vi "THETA_2.vi"(8 "error in (no error)":errorcluster, 11 "reference in":refnum<class "Manipulator.lvclass">) -> (0 "error out":errorcluster, 3 "reference out":refnum<class "Manipulator.lvclass">)   [LabVIEW 2014, in "Manipulator.lvclass"]
uses:
  Manipulator.lvclass
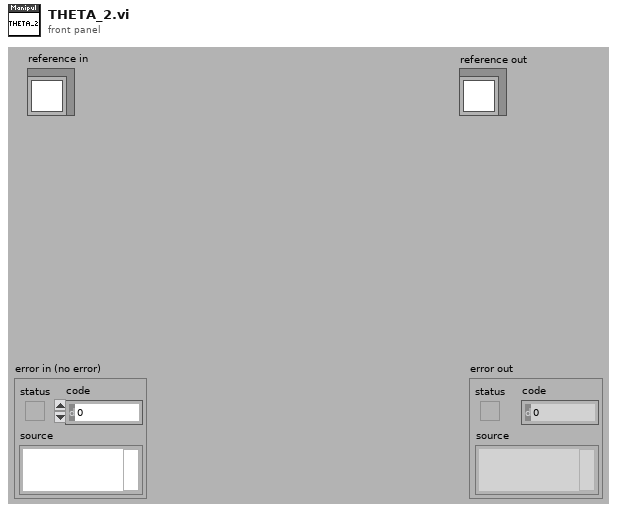
[diagram p1: front panel]
types:
  T1 = typedef "Manipulator.lvclass/ObjectAttributes.ctl" = cluster{"Coordinates":cluster{"X":dbl, "Y":dbl, "Z":dbl}, "Angles":cluster{"THETA_1":dbl, "THETA_2":dbl, "THETA_3":dbl, "THETA_4":dbl, "THETA_5":dbl, "THETA_6":dbl, "THETA_7":dbl, "THETA_8":dbl, "THETA_9":dbl, "THETA_10":dbl}, "Lengths":cluster{"a":dbl, "b":dbl, "c":dbl, "d":dbl, "e":dbl}}
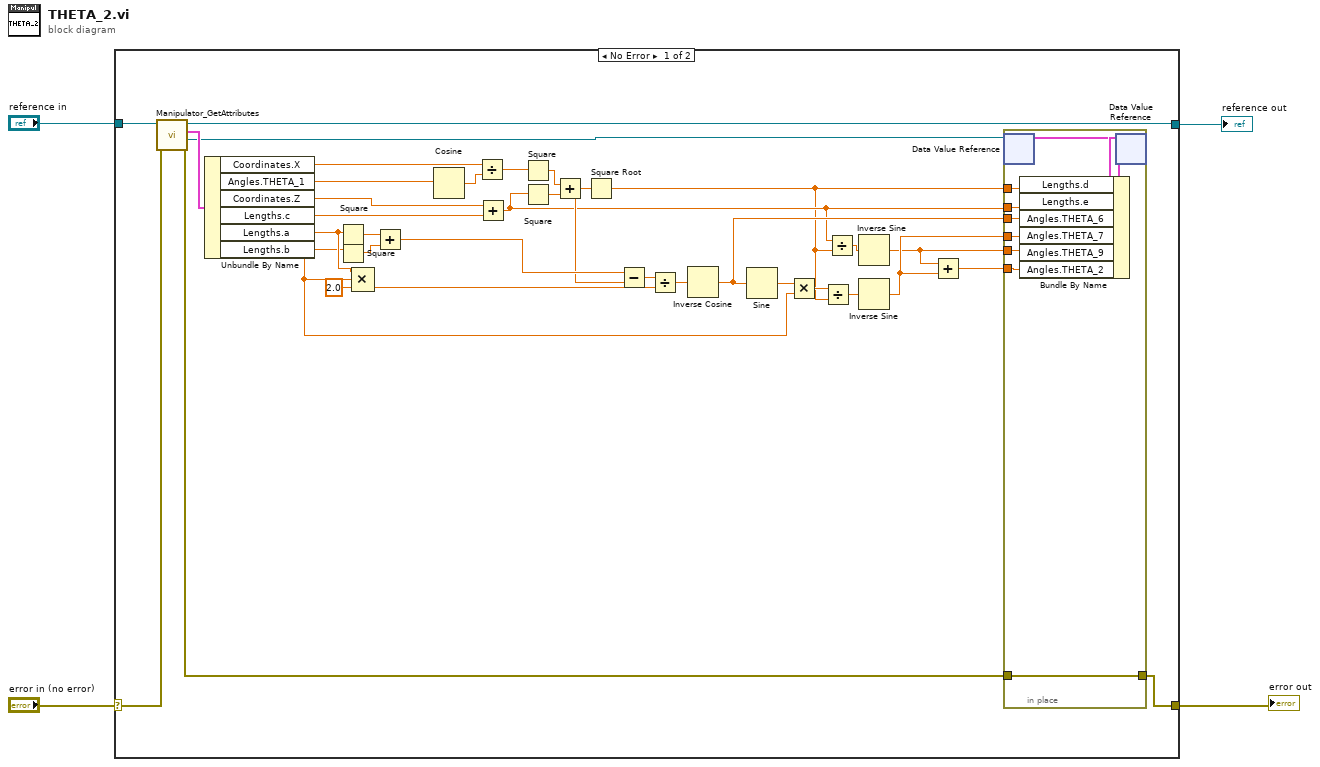
[diagram p0: block diagram]
diagram:
  n1 = case shown="No Error" "error in (no error)" {
    selector: "error in (no error)" -> [w38 w50]
    tunnel: [w11 w50] -> w3
    tunnel: [w36 w49] -> w1
    tunnel: "reference in" -> [w39 w49]
    frame No Error {
      n2 = call "Manipulator_GetAttributes.vi"("error in (no error)"=w38, "reference in"=w39) -> ("error out"=w34:errorcluster, "DataRef"=w35:refnum<data-value>, "Data"=w37:T1, "reference out"=w36:refnum<class "Manipulator.lvclass">)  [unwired: 6 in]
      n3 = Unbundle By Name(w37) -> ("Coordinates.X"=w33:dbl, "Angles.THETA_1"=w27:dbl, "Coordinates.Z"=w31:dbl, "Lengths.c"=w26:dbl, "Lengths.a"=w20:dbl, "Lengths.b"=w14:dbl)
      n4 = Square(x=w20) -> (x^2=w25:dbl)
      n5 = Square(x=w14) -> (x^2=w24:dbl)
      n6 = Compound Arithmetic op=MULTIPLY(w20, w14, 2.0 ("value")) -> (w18:dbl)
      n7 = Add(x=w25, y=w24) -> (x+y=w23:dbl)
      n8 = Cosine(x=w27) -> (cos(x)=w32:dbl)
      n9 = Divide(x=w33, y=w32) -> (x/y=w28:dbl)
      n10 = Add(x=w31, y=w26) -> (x+y=w9:dbl)
      n11 = Square(x=w28) -> (x^2=w30:dbl)
      n12 = Square(x=w9) -> (x^2=w29:dbl)
      n13 = Add(x=w30, y=w29) -> (x+y=w22:dbl)
      n14 = Square Root(x=w22) -> (sqrt(x)=w8:dbl)
      n15 = Subtract(x=w23, y=w22) -> (x-y=w21:dbl)
      n16 = Divide(x=w21, y=w18) -> (x/y=w17:dbl)
      n17 = Inverse Cosine(1:w17) -> (0:w16:dbl)
      n18 = Sine(x=w16) -> (sin(x)=w15:dbl)
      n19 = Multiply(x=w15, y=w14) -> (x*y=w13:dbl)
      n20 = Divide(x=w13, y=w8) -> (x/y=w12:dbl)
      n21 = Divide(x=w9, y=w8) -> (x/y=w10:dbl)
      n22 = Inverse Sine(1:w10) -> (0:w6:dbl)
      n23 = Inverse Sine(1:w12) -> (0:w7:dbl)
      n24 = Add(x=w6, y=w7) -> (x+y=w5:dbl)
      n25 = in-place {
        in-place-border: w34 -> [w48]
        in-place-border: [w48] -> w11
        in-place-border: w8 -> [w45]
        in-place-border: w9 -> [w44]
        in-place-border: w16 -> [w43]
        in-place-border: w7 -> [w42]
        in-place-border: w6 -> [w41]
        in-place-border: w5 -> [w40]
        n26 = in-place-dvr #1(w35) -> (w46:T1)  [unwired: 1 out]
        n27 = Bundle By Name(cluster=w46, "Lengths.d"=w45, "Lengths.e"=w44, "Angles.THETA_6"=w43, "Angles.THETA_7"=w42, "Angles.THETA_9"=w41, "Angles.THETA_2"=w40) -> (w47:T1)
        n28 = in-place-dvr #1(w47) -> ()  [unwired: 2 out]
      }
    }
    frame Error {
    }
  }
  "error out" <- w3
  "reference out" <- w1
